vi "AttrMapToCluster.vi"(8 "error in (no error)":errorcluster, 11 "AttrMap":T1) -> (0 "error out":errorcluster, 3 "Cluster":variant)   [LabVIEW 2019]
uses:
  Typedef/Def-AttrMap.ctl
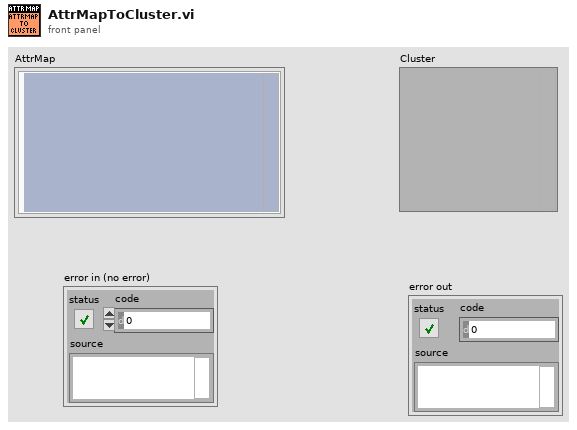
[diagram p1: front panel]
types:
  T1 = typedef "Def-AttrMap.ctl" = cluster{"Map":variant}
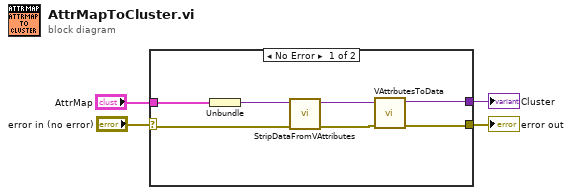
[diagram p0: block diagram]
diagram:
  n1 = case shown="No Error" "error in (no error)" {
    selector: "error in (no error)" -> [w6 w12]
    tunnel: [w9 w12] -> w4
    tunnel: "AttrMap" -> [w11 _]
    tunnel: [w8 _] -> w1
    frame No Error {
      n2 = Unbundle(w11) -> ("Map"=w10:variant)
      n3 = call "StripDataFromVAttributes.vi"("error in (no error)"=w6, "Map"=w10) -> ("error out"=w5:errorcluster, "duplicate variant"=w7:variant)  [unwired: 8 in]
      n4 = call "VAttrbutesToData.vi"("error in (no error)"=w5, "VAttributes"=w7) -> ("error out"=w9:errorcluster, "data"=w8:variant)  [unwired: 8 in]
    }
    frame Error {
    }
  }
  "Cluster" <- w1
  "error out" <- w4
